vi "GetInitGyroOffset.vi"(3 "NXT":T1={"error"={"status"=FALSE, "code"=0, "source"=""}, "address"="", "NXT #"=-1, "Show Error"=TRUE, "Connection"=4} {"Connection" items=["USB", "Bluetooth", "USB then Bluetooth", "Last Connection", "Preference"]}) -> (0 "GyroOffset":sgl, 1 "NXT 2":T1={"error"={"status"=FALSE, "code"=0, "source"=""}, "address"="", "NXT #"=-1, "Show Error"=TRUE, "Connection"=4} caption="NXT" {"Connection" items=["USB", "Bluetooth", "USB then Bluetooth", "Last Connection", "Preference"]})   [LabVIEW 2009]
uses:
  <vilib>/NXT/Subs/LVHSConnector.ctl
  <vilib>/NXT/HiTechnic/Sensors/HiTechnic Port.ctl
  <vilib>/NXT/Block Support/NXT_InputPort.ctl
panel:
  # "HTWay - GetInitGyroOffset\nCalculates an initial Gyro Offset.  Takes the average of 100 samples but will\nreject and resample if the max of all samples is more than 1 from the average."
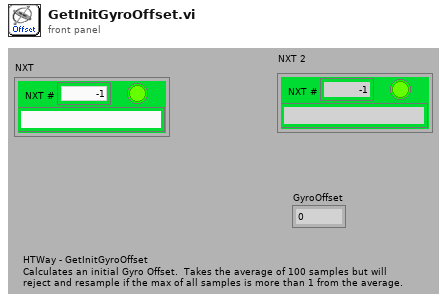
[diagram p1: front panel]
types:
  T1 = typedef "LVHSConnector.ctl" = cluster{"error":errorcluster, "address":string, "NXT #":i32, "Show Error":bool, "Connection":u16}
  T2 = typedef "HiTechnic Port.ctl" = cluster{"Port":T3, "MUX Port":u8}
  T3 = typedef "NXT_InputPort.ctl" = u8
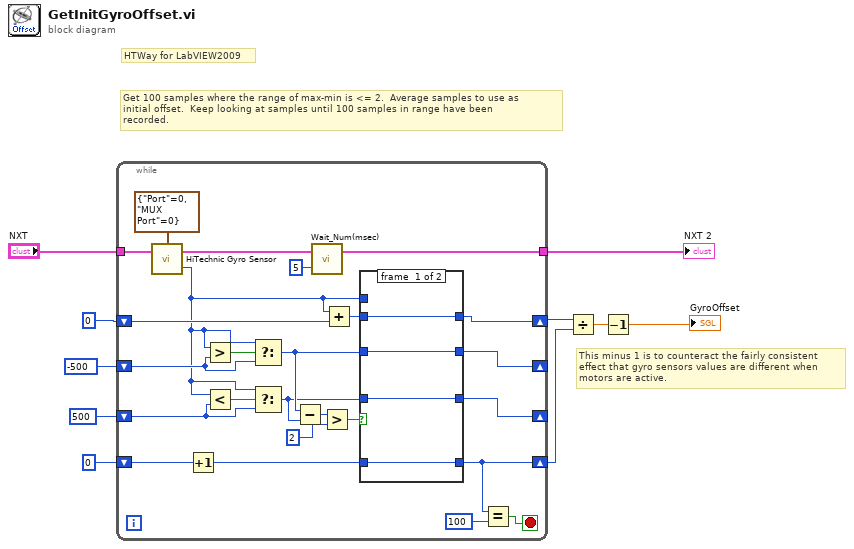
[diagram p0: block diagram]
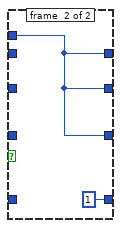
[diagram p2: hidden frame]
diagram:
  # "This minus 1 is to counteract the fairly consistent\neffect that gyro sensors values are different when\nmotors are active."
  # "Get 100 samples where the range of max-min is <= 2.  Average samples to use as\ninitial offset.  Keep looking at samples until 100 samples in range have been \nrecorded."
  # "HTWay for LabVIEW2009"
  n1 = while {
    shift-right: [w27] -> _
    shift-left: i16 -500 ("Gyro Value") -> [w32]
    shift-right: [w26] -> _
    shift-left: i16 500 ("Gyro Value") -> [w31]
    shift-right: [w17] -> w2
    shift-left: i16 0 ("Gyro Value") -> [w20]
    shift-right: [w22] -> w3
    shift-left: i16 0 ("Gyro Value") -> [w23]
    tunnel: "NXT" -> [w13]
    tunnel: [w12] -> w4
    stop <- w18 stop-if-true
    n2 = call <vilib>:"HiTechnic Gyro Sensor.vi"("NXT"=w13, "Port/MUX"=T2 {"Port"=0, "MUX Port"=0}) -> ("Gyro Value"=w11:i16, "NXT"=w15:T1)  [unwired: 1 in]
    n3 = Increment(x=w20) -> (x+1=w19:i16)
    n4 = Greater?(x=w11, y=w32) -> (0:w34:bool)
    n5 = Less?(x=w11, y=w31) -> (x < y?=w33:bool)
    n6 = Select(t=w11, s=w34, f=w32) -> (s? t:f=w25:i16)
    n7 = Select(t=w11, s=w33, f=w31) -> (s? t:f=w24:i16)
    n8 = Subtract(x=w25, y=w24) -> (x-y=w30:i16)
    n9 = call <vilib>:"Wait_Num(msec).vi"("Time (100 msec)"=u32 5, "NXT"=w15) -> ("NXT"=w12:T1)  [unwired: 2 in]
    n10 = Greater?(x=w30, y=i16 2) -> (0:w28:bool)
    n11 = Add(x=w11, y=w23) -> (x+y=w21:i16)
    n12 = case shown="True" w28 {
      tunnel: [w39 w40] -> w27
      tunnel: w11 -> [_ w40]
      tunnel: [w38 w40] -> w26
      tunnel: w25 -> [w39 _]
      tunnel: w24 -> [w38 _]
      tunnel: [w37 i16 1 ("Gyro Value")] -> w17
      tunnel: w19 -> [w37 _]
      tunnel: [w36 w40] -> w22
      tunnel: w21 -> [w36 _]
      frame #0 {
      }
      frame #1 {
      }
    }
    n13 = Equal?(x=w17, y=i16 100) -> (x = y?=w18:bool)
  }
  "NXT 2" <- w4
  n14 = Divide(x=w3, y=w2) -> (x/y=w1:dbl)
  n15 = Decrement(x=w1) -> (x-1=→"GyroOffset":dbl)
